vi "TestModelingLoop.vi"() -> (0 "Cur_stdv":dbl=50.0, 1 "BErr":dbl format="%.2f", 2 "SNR":dbl format="%#_13g")   [LabVIEW 2014]
uses:
  <vilib>/Simulation/Scripting/Companion Diagram/SimConfigNode/SimParams.ctl
  <vilib>/Simulation/Scripting/Companion Diagram/SimConfigNode/_simSolvers.ctl
  <vilib>/Simulation/Implementation/Shared/SIMSCR Execution Mode.ctl
  <vilib>/Simulation/Param Hierarchy/Typedefs/SIMPH Param Control Actions.ctl
  <vilib>/Simulation/Implementation/Shared/NILVSim_ParamChanged.vi
  <vilib>/Simulation/Implementation/Shared/NILVSIM_BeginStep.vi
  <vilib>/Simulation/Utility/Implementation/NILVSim Memory.llb/NILVSim Memory (core).vi
  <vilib>/Simulation/Implementation/Shared/NILVSim_Manager.vi
  <vilib>/Utility/error.llb/Clear Errors.vi
  <vilib>/Simulation/Implementation/Shared/NILVSim_FinalizeModel.vi
  <vilib>/Simulation/Implementation/Shared/SIM Unbundle Sim Info.vi
  <vilib>/Simulation/Implementation/Shared/NILVSim_Initialize.vi
  <vilib>/ptbypt/Signal Generation.llb/Gaussian White Noise PtByPt.vi
  MessageCorrect.vi
  <vilib>/Simulation/Utility/Implementation/NILVSim Get Time and IsAcceptedStep.vi
  <vilib>/gmath/statdist.llb/Correlation Coefficient.vi
  SNR.vi
  <vilib>/Simulation/Implementation/Shared/SIMSH Read Queue.vi
  <vilib>/Simulation/Implementation/Shared/NILVSim_GetModelError.vi
  <vilib>/Simulation/Implementation/Shared/SIM Bundle Sim Info.vi
  <vilib>/Simulation/Scripting/Companion Diagram/SimConfigNode/SimDog.xnode
  <vilib>/Simulation/Implementation/XNodeFramework/SimXNode/SimX.xnode
  <vilib>/Simulation/EMI/Plugins/Multisim Design/MultisimEMICtrl.dll
  <vilib>/ptbypt/NI_PtbyPt.lvlib
  <vilib>/gmath/NI_Gmath.lvlib
  <vilib>/Simulation/Implementation/Shared/NI_SIM_Implementation.lvlib
panel:
  in  "STDV":dbl[](array[numeric])=[1.0, 1.0, 1.0]
  out "SNR 2":dbl[](array[numeric])
  out "BER@":dbl[](array[numeric])
  in  "X 3":dbl[](array[numeric])=[1.0, 1.0, 1.0]
  out "Timer":i32
  out "Correlation":T1(graph)={"correlation coefficient r"=-0.6285527240782425, "h 2"=0.0}
  out "Input Signal":dynamicdata(graph)
  out "Cur_size":i32=24
  in  "Time_code":dbl=0.002
  in  "h_mod":dbl=1e-06
  out "Message size":i32=24
  out "AttractorSynch":dynamicdata(graph)=[{"t0"=timestamp(3822748401.3125644 s since 1904-01-01), "dt"=1.0, "Y"=array[2000 elements], "attributes"=variant("NI_ChannelName"=variant(string "Collected"))}]
  out "AttractorBase":dynamicdata(graph)=[{"t0"=timestamp(3822748401.3125644 s since 1904-01-01), "dt"=1.0, "Y"=array[2000 elements], "attributes"=variant("NI_ChannelName"=variant(string "Collected"))}]
  out "Recive":bool[](array[boolean])=[FALSE, TRUE, TRUE, TRUE, TRUE, FALSE, TRUE, FALSE, TRUE, FALSE, TRUE, FALSE, TRUE, FALSE, TRUE, FALSE, FALSE, TRUE, FALSE, TRUE, TRUE, FALSE, FALSE, FALSE]
  out "Model":dbl=500.00000000000006
  out "cos":dbl=0.8270710623015505
  out "sin":dbl=-1.266949846684384
  in  "K":dbl=97.0
  in  "X 2":dbl[](array[numeric])=[1.0, 1.0, 1.0]
  out "Noise":dynamicdata(graph)
  out "Sending":bool
  out "Clear":dynamicdata(graph)
  in  "X":dbl[](array[numeric])=[0.1, 0.1, 0.1]
  in  "A":dbl[](array[numeric])=[10.0, 28.0, 2.666666]
  in  "h_CD":dbl=0.006
  out "Send":bool[](array[boolean])=[TRUE, FALSE, FALSE, FALSE, TRUE, TRUE, FALSE, FALSE, FALSE, TRUE, FALSE, FALSE, TRUE, TRUE, FALSE, FALSE, TRUE, TRUE, FALSE, FALSE, TRUE, TRUE, FALSE, FALSE]
  in  "Input string":string="123"
  # "Chaos theory examines how tiny changes in initial conditions can result in vastly different outcomes in complex systems. This unpredictability appears in weather, ecosystems, and financial markets."
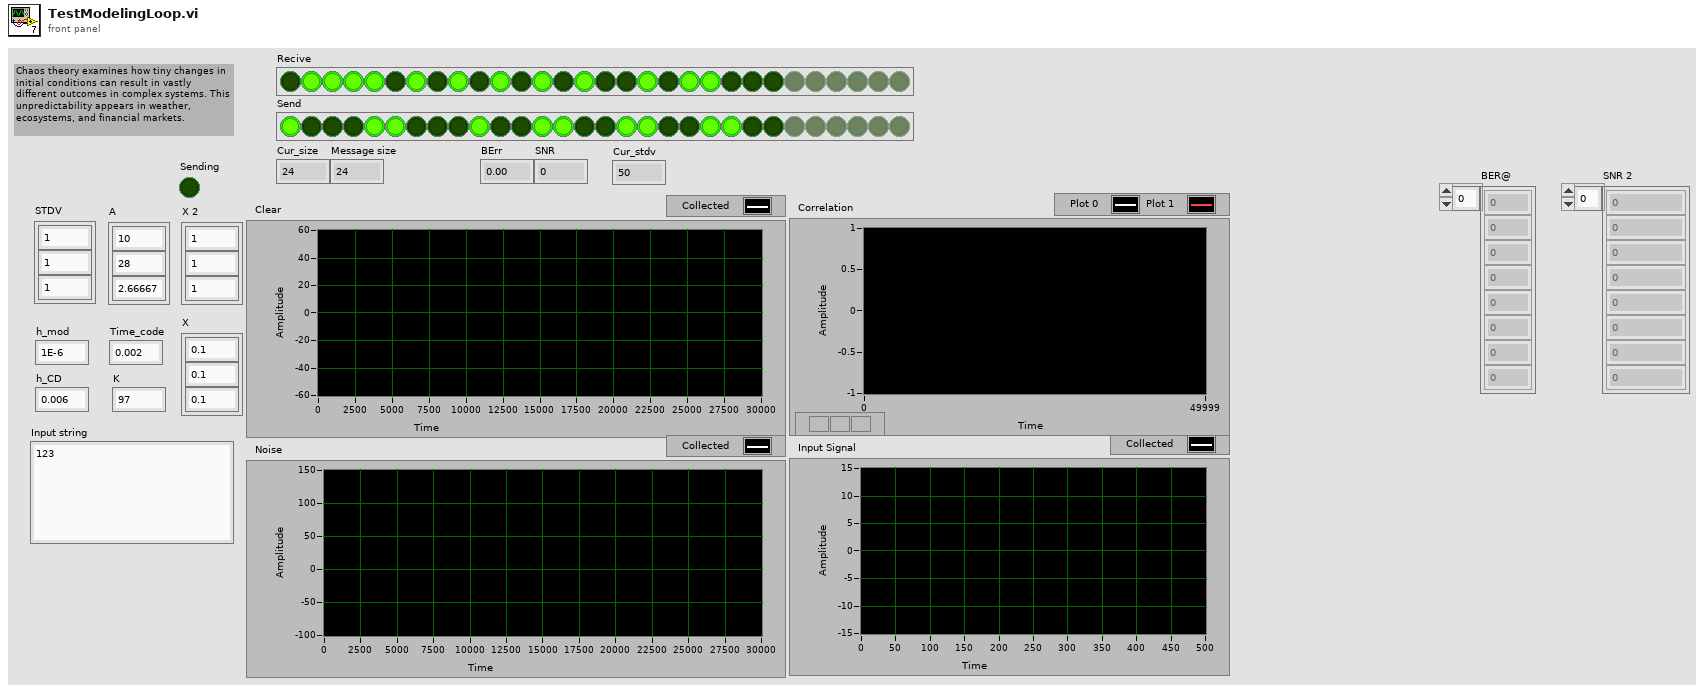
[diagram p1: front panel]
types:
  T1 = cluster{"correlation coefficient r":dbl, "h 2":dbl}
  T2 = typedef "SIMSCR Execution Mode.ctl" = enum16{"Simulate to Completion", "Single Time-Step Simulation (Fixed Step Only)"}
  T3 = typedef "SIMPH Param Control Actions.ctl" = enum16{"get params", "set params"}
  T4 = typedef "SimParams.ctl" = cluster{"Initial Time (s)":dbl, "Final Time (s)":dbl, "Step Size (s)":dbl, "ODE Solver":T5, "Minimum Step Size (s)":dbl, "Maximum Step Size (s)":dbl, "Relative Tolerance":dbl, "Absolute Tolerance":dbl, "Software Timing":bool, "Initial Step Size (s)":dbl, "Automatic Fixed Step Size?":bool, "Automatic Discrete Step Size?":bool, "Discrete Step Size (s)":dbl, "Calculate using Time Step":bool, "Solver Wired?":bool, "Prev.Frm.Expected End":u64, "Prev.Frm.Actual End":u64, "Prev.Frm.Finished Late?":bool, "Prev.Iter.Expected End":u64, "Prev.Iter.Actual End":u64, "Prev.Iter.Finished Late?":bool, "Expected Iteration Start":u64, "Actual Iteration Start":u64, "Expected Frame Start":u64, "Actual Frame Start":u64, "Source Name":string, "Name":string, "Period":i64, "Deadline":i64, "Offset":i64, "Start":i64, "Priority":i32, "Timeout":i32, "Processor":i32, "Mode":enum32{"No Change", "Process missed periods, maintain original phase", "Discard missed periods, maintain original phase", "Process missed periods, ignore original phase", "Discard missed periods, ignore original phase"}, "Wakeup reason":enum32{"Normal", "Aborted", "Asynchronous wakeup", "Timing source error", "Timed loop error", "Timeout"}, "Error":errorcluster, "Source Type":string, "Secondary Source Type":string, "Global End Time":u64, "Global Start Time":u64, "Full Solver Reset":bool, "Execution Mode":T2, "Nan/Inf Check":bool, "Custom Solver Library":string, "Solver Is Variable":bool, "custom solver name":string, "Signal Collection Decimation":u32}
  T5 = typedef "_simSolvers.ctl" = enum16{"Runge-Kutta 1 (Euler)", "Runge-Kutta 2", "Runge-Kutta 3", "Runge-Kutta 4", "Runge-Kutta 23 (variable)", "Runge-Kutta 45 (variable)", "BDF (variable)", "Adams-Moulton (variable)", "Rosenbrock (variable)", "Discrete States Only", "SDIRK 4 (variable)", "Radau 5 (variable)", "Radau 9 (variable)", "Radau 13 (variable)", "Radau [Variable Order] (variable)", "Gear's Method (variable)", "Linearizer", "State Query", "Trim Eval", "Custom Solver"}
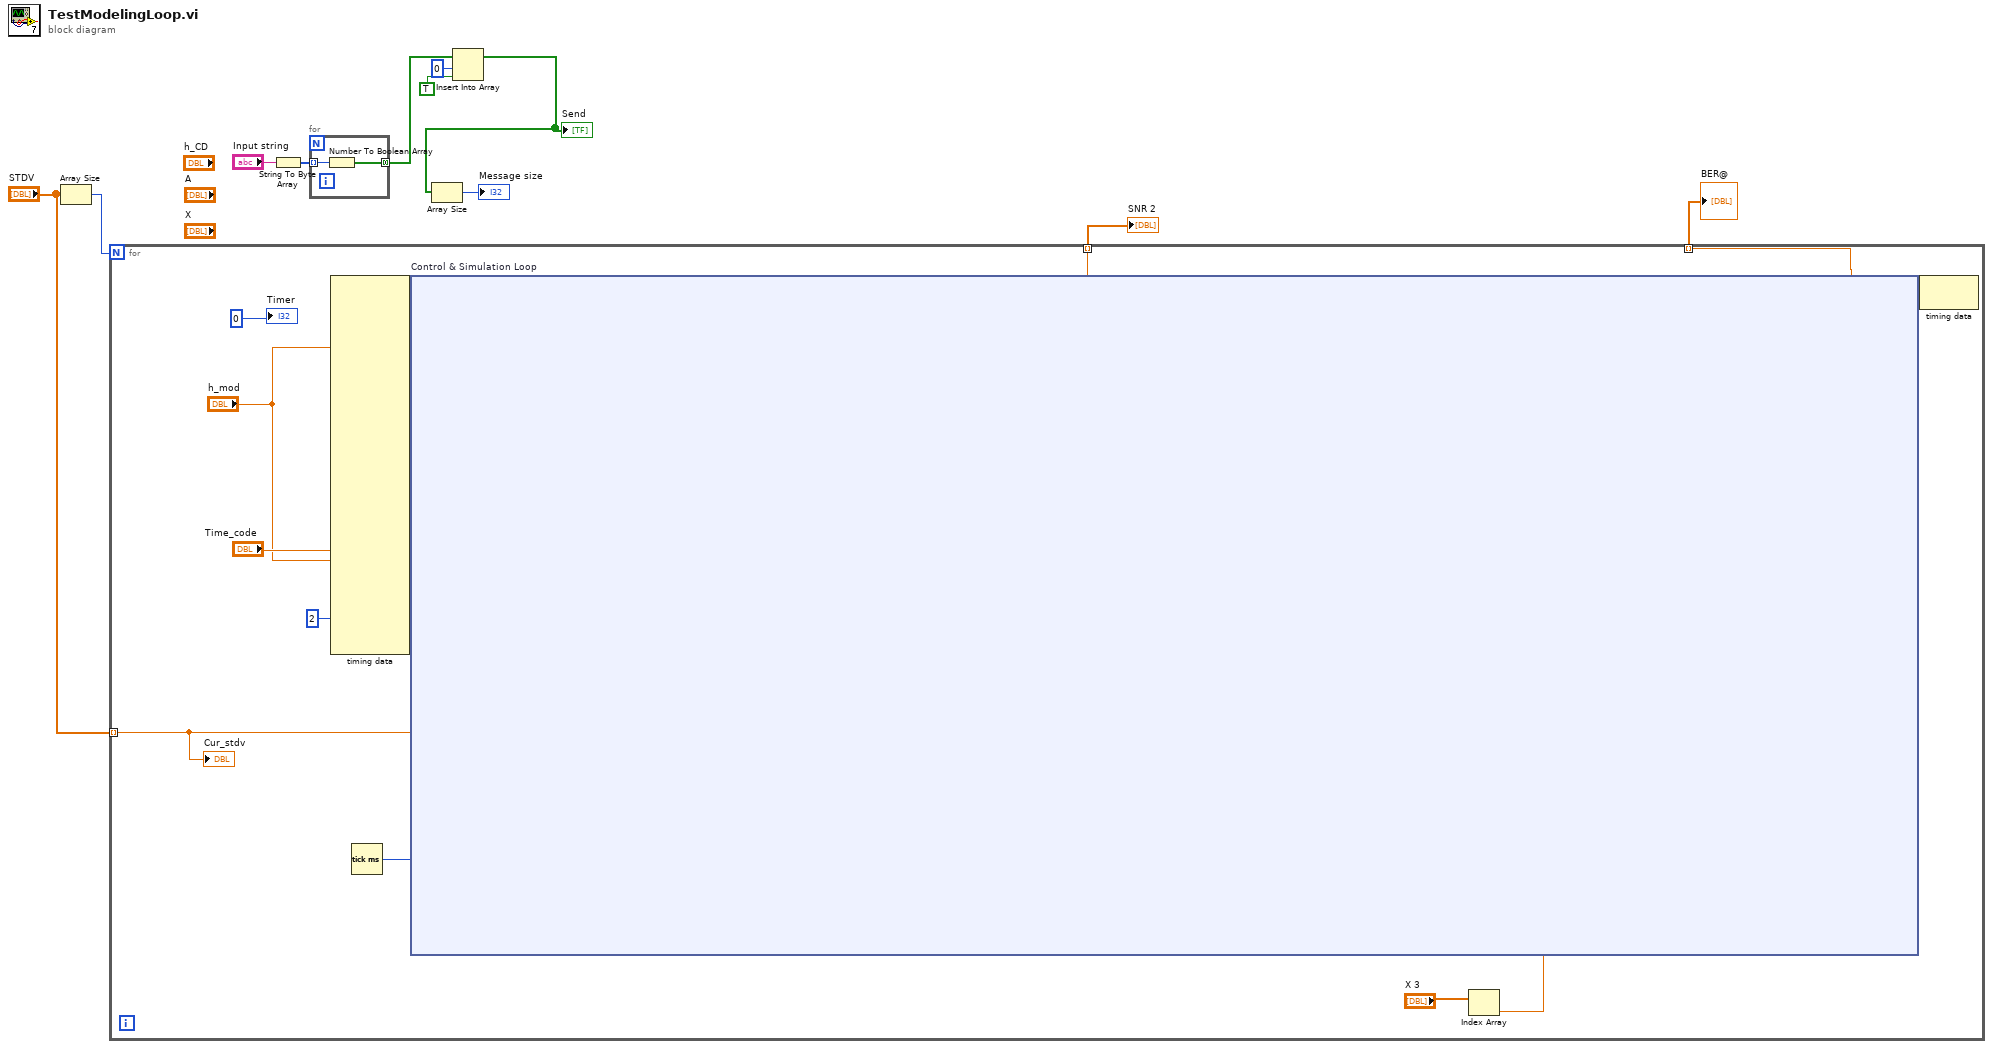
[diagram p0: block diagram]
diagram:
  n1 = Array Size(array="STDV") -> (size(s)=w2:i32)
  n2 = for {
    N: w2 -> [_]
    tunnel: [w17] -> w4 mode=indexing
    tunnel: [w16] -> w3 mode=indexing
    tunnel: "STDV" -> [w13] mode=indexing
    n3 = node-c288("h_mod", 2) -> (w23:variant)  [unwired: 22 in]
    n4 = Tick Count (ms)() -> (millisecond timer value=w18:u32)
    n5 = Index Array(array="X 3") -> (element=w20:dbl)  [unwired: 1 in]
    n6 = node-c254 "Control & Simulation Loop"(w23, w13, "Time_code", "h_mod", w20, w18) -> (w22:variant, w17:dbl, w16:dbl)
    n7 = node-c288(w22) -> ()  [unwired: 1 out]
    "Cur_stdv" <- w13
    "Timer" <- 0 ("Constant 7")
  }
  "BER@" <- w4
  "SNR 2" <- w3
  n8 = String To Byte Array(string="Input string") -> (unsigned byte array=w11:u8[])
  n9 = for {
    tunnel: w11 -> [w860] mode=indexing
    tunnel: [w859] -> w8 mode=concatenating
    n10 = Number To Boolean Array(number=w860) -> (Boolean array=w859:bool[])
  }
  n11 = Insert Into Array(array=w8, index=0, new element=TRUE ("Constant 2")) -> (w5:bool[])
  "Send" <- w5
  n12 = Array Size(array=w5) -> (size(s)=→"Message size":i32)
